vi "GetOvalWidth.vi"(8 "error in (no error)":errorcluster, 11 "RoundRectangle in":refnum<class "RoundRectangle.lvclass">) -> (0 "error out":errorcluster, 2 "Oval Width":i16, 3 "RoundRectangle out":refnum<class "RoundRectangle.lvclass">)   [LabVIEW 2021, in "Picture2D.lvlib" / "RoundRectangle.lvclass"]
uses:
  RoundRectangle.lvclass
  RoundRectangle.lvclass/RoundRectangle.ctl
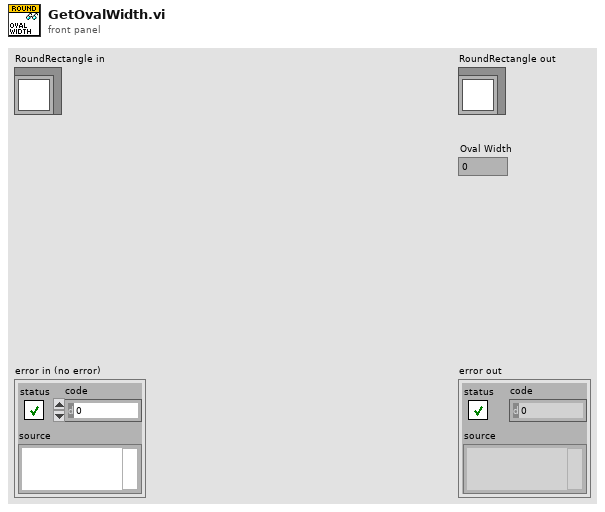
[diagram p1: front panel]
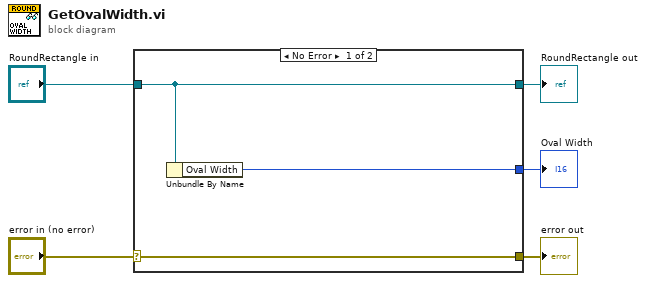
[diagram p0: block diagram]
diagram:
  n1 = case shown="No Error" "error in (no error)" {
    selector: "error in (no error)" -> [w8 w9]
    tunnel: [w8 w9] -> w4
    tunnel: [w7 w10] -> w2
    tunnel: "RoundRectangle in" -> [w7 w10]
    tunnel: [w6 _] -> w1
    frame No Error {
      n2 = Unbundle By Name(w7) -> ("Oval Width"=w6:i16)
    }
    frame Error {
    }
  }
  "error out" <- w4
  "RoundRectangle out" <- w2
  "Oval Width" <- w1
